vi "Read Measurement (Third Order Intercept).vi"(0 "VISA resource name":refnum<visa-resource-name>, 5 "TOI Output Format (1)":i32=1 min=0 max=2 step=1, 11 "error in (no error)":errorcluster) -> (4 "VISA resource name out":refnum<visa-resource-name>, 6 "TOI Output Format1":dbl[](array[numeric]), 8 "TOI Output Format2":T2 {"Upper_TOI" format="%.2f"; "Lower_TOI" format="%.2f"; "Worst_TOI" format="%.2f"}, 10 "TOI Output Format3":T1 {"worst_TOI" format="%.2f"; "worst_Rel" format="%.3f"; "worst_Amp" format="%.2f"; "Upper_TOI" format="%.2f"; "Upper_3rd_Rel" format="%.3f"; "Upper_3rd_Amp" format="%.2f"; "Lower_TOI" format="%.2f"; "Lower_3rd_Rel" format="%.3f"; "Upper_Tone_Amp" format="%.2f"; "Lower_Tone_Amp" format="%.2f"; "Lower_3rd_Amp" format="%.2f"}, 15 "error out":errorcluster)   [LabVIEW 2020, in "Anritsu Signal Analyzer Series.lvlib"]
doc: "Reads the measurement result of the TOI measurement."
uses:
  Anritsu Signal Analyzer Series.lvlib
panel:
  # "Frequency(Hz)"
  # "Amp(dBm)"
  # "Relative(dBc)"
  # "TOI(dBm)"
  # "Lower 3rd"
  # "Lower Tone"
  # "Upper Tone"
  # "Upper 3rd"
  # "TOI Worst"
  # "TOI(dBm)"
  # "Frequency(Hz)"
  # "Worst"
  # "Lower"
  # "Upper"
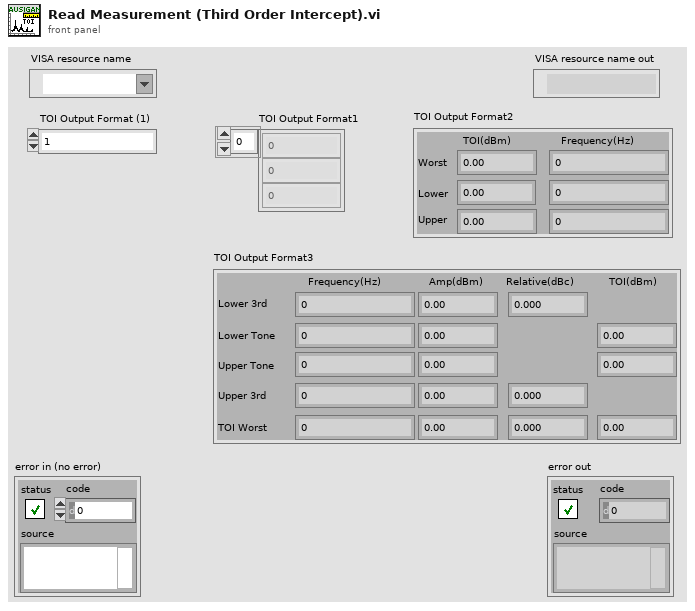
[diagram p1: front panel]
types:
  T1 = cluster{"Lower_3rd_Freq":dbl, "Lower_3rd_Amp":dbl, "Lower_3rd_Rel":dbl, "Lower_Tone_Freq":dbl, "Lower_Tone_Amp":dbl, "Lower_TOI":dbl, "Upper_Tone_Freq":dbl, "Upper_Tone_Amp":dbl, "Upper_TOI":dbl, "Upper_3rd_Freq":dbl, "Upper_3rd_Amp":dbl, "Upper_3rd_Rel":dbl, "worst_TOI_Freq":dbl, "worst_Amp":dbl, "worst_Rel":dbl, "worst_TOI":dbl}
  T2 = cluster{"Worst_TOI":dbl, "Worst_TOI_Freq":dbl, "Lower_TOI":dbl, "Lower_3rd_Freq":dbl, "Upper_TOI":dbl, "Upper_3rd_Freq":dbl}
  T3 = cluster{"Lower_3rd_Freq":dbl, "Lower_3rd_Amp":dbl, "Lower_3rd_Rel":dbl, "Lower_3rd_TOI":dbl, "Lower_Tone_Freq":dbl, "Lower_Tone_Amp":dbl, "Upper_Tone_Freq":dbl, "Upper_Tone_Amp":dbl, "Upper_3rd_Freq":dbl, "Upper_3rd_Amp":dbl, "Upper_3rd_Rel":dbl, "Upper_3rd_TOI":dbl, "worst_TOI_Freq":dbl, "worst_Amp":dbl, "worst_Rel":dbl, "worst_TOI":dbl}
  T4 = cluster{"_Default":dbl, dbl, "_Default":dbl, dbl, "_Default":dbl, dbl}
  T5 = cluster{"_Default":dbl, "_Default":dbl, "_Default":dbl, "_Default":dbl, "_Default":dbl, "_Default":dbl}
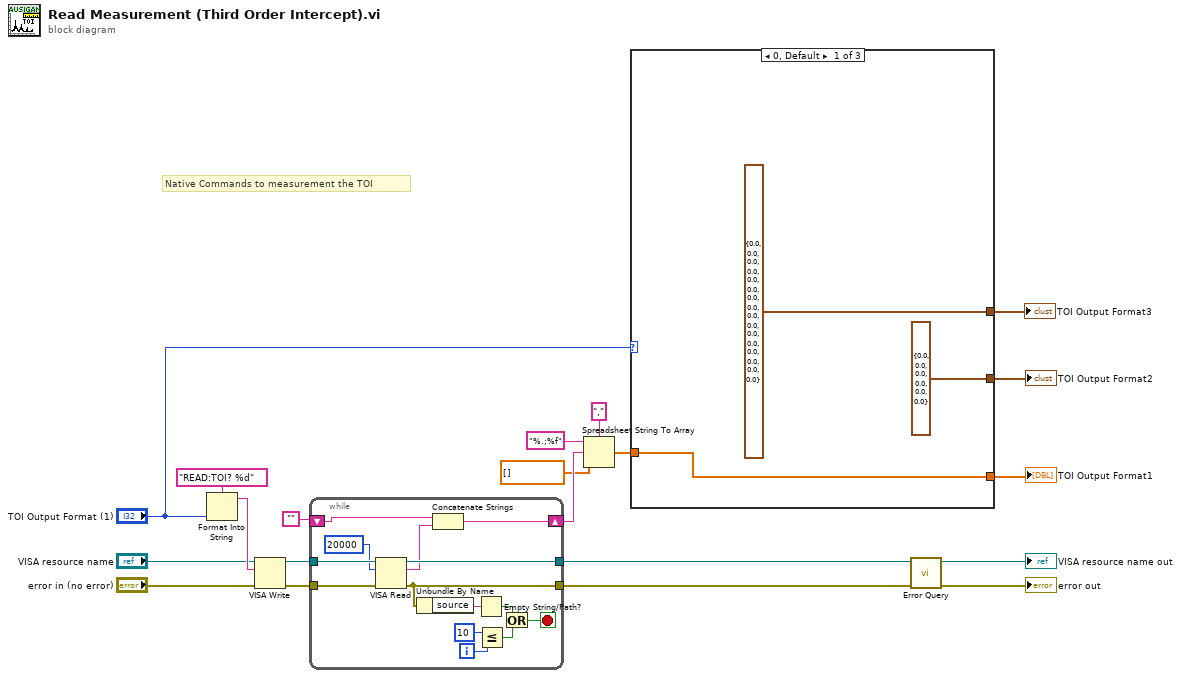
[diagram p0: block diagram]
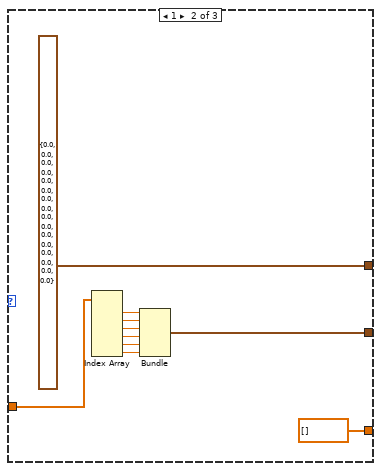
[diagram p2: hidden frame]
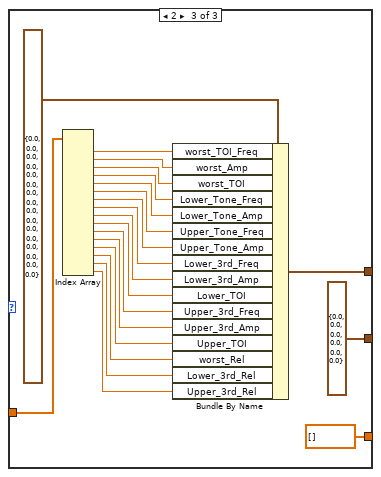
[diagram p3: hidden frame]
diagram:
  # "Native Commands to measurement the TOI"
  n1 = Format Into String(format string="READ:TOI? %d" ("_Command"), "TOI Output Format (1)") -> (resulting string=w3:string)  [unwired: 2 in, 1 out]
  n2 = VISA Write(VISA resource name="VISA resource name", write buffer=w3, error in (no error)="error in (no error)") -> (VISA resource name out=w9:refnum<visa-resource-name>, error out=w10:errorcluster)  [unwired: 1 out]
  n3 = while {
    tunnel: w9 -> [w34]
    tunnel: w10 -> [w33]
    tunnel: [w31] -> w4
    tunnel: [w30] -> w5
    shift-right: [w29] -> w11
    shift-left: "" -> [w27]
    i -> [w22]
    stop <- w26 stop-if-true
    n4 = VISA Read(VISA resource name=w34, byte count=u32 20000 ("byte count (0)"), error in (no error)=w33) -> (VISA resource name out=w31:refnum<visa-resource-name>, read buffer=w28:string, error out=w30:errorcluster)  [unwired: 1 out]
    n5 = Unbundle By Name(w30) -> ("source"=w25:string)
    n6 = Concatenate Strings(w27, w28) -> (w29:string)
    n7 = Empty String/Path?(string/path=w25) -> (empty?=w21:bool)
    n8 = Less Or Equal?(x=10, y=w22) -> (x <= y?=w24:bool)
    n9 = Or(x=w21, y=w24) -> (x .or. y?=w26:bool)
  }
  n10 = Spreadsheet String To Array(delimiter (Tab)=",", format string="%.;%f" ("Format String"), spreadsheet string=w11, array type (2D Dbl)=dbl[] []) -> (array=w14:dbl[])
  n11 = case shown="0, Default" "TOI Output Format (1)" {
    tunnel: w14 -> [w37 w46 w56]
    tunnel: [w37 dbl[] [] dbl[] []] -> w17
    tunnel: [T4 {"_Default"=0.0, 0.0, "_Default"=0.0, 0.0, "_Default"=0.0, 0.0} w42 T4 {"_Default"=0.0, 0.0, "_Default"=0.0, 0.0, "_Default"=0.0, 0.0}] -> w16
    tunnel: [T3 {"Lower_3rd_Freq"=0.0, "Lower_3rd_Amp"=0.0, "Lower_3rd_Rel"=0.0, "Lower_3rd_TOI"=0.0, "Lower_Tone_Freq"=0.0, "Lower_Tone_Amp"=0.0, "Upper_Tone_Freq"=0.0, "Upper_Tone_Amp"=0.0, "Upper_3rd_Freq"=0.0, "Upper_3rd_Amp"=0.0, "Upper_3rd_Rel"=0.0, "Upper_3rd_TOI"=0.0, "worst_TOI_Freq"=0.0, "worst_Amp"=0.0, "worst_Rel"=0.0, "worst_TOI"=0.0} ("TOI(2)") T1 {"Lower_3rd_Freq"=0.0, "Lower_3rd_Amp"=0.0, "Lower_3rd_Rel"=0.0, "Lower_Tone_Freq"=0.0, "Lower_Tone_Amp"=0.0, "Lower_TOI"=0.0, "Upper_Tone_Freq"=0.0, "Upper_Tone_Amp"=0.0, "Upper_TOI"=0.0, "Upper_3rd_Freq"=0.0, "Upper_3rd_Amp"=0.0, "Upper_3rd_Rel"=0.0, "worst_TOI_Freq"=0.0, "worst_Amp"=0.0, "worst_Rel"=0.0, "worst_TOI"=0.0} ("TOI Output Format3") w57] -> w15
    frame 0, Default {
    }
    frame 1 {
      n12 = Index Array(array=w46) -> (element #1=w45:dbl, element #2=w41:dbl, element #3=w44:dbl, element #4=w40:dbl, element #5=w43:dbl, element #6=w39:dbl)  [unwired: 6 in]
      n13 = Bundle("_Default"=w45, "_Default"=w41, "_Default"=w44, "_Default"=w40, "_Default"=w43, "_Default"=w39) -> (w42:T5)  [unwired: 1 in]
    }
    frame 2 {
      n14 = Index Array(array=w56) -> (element #1=w49:dbl, element #2=w58:dbl, element #3=w59:dbl, element #4=w50:dbl, element #5=w60:dbl, element #6=w51:dbl, element #7=w61:dbl, element #8=w52:dbl, element #9=w62:dbl, element #10=w63:dbl, element #11=w53:dbl, element #12=w64:dbl, element #13=w65:dbl, element #14=w66:dbl, element #15=w67:dbl, element #16=w68:dbl)  [unwired: 16 in]
      n15 = Bundle By Name(cluster=T1 {"Lower_3rd_Freq"=0.0, "Lower_3rd_Amp"=0.0, "Lower_3rd_Rel"=0.0, "Lower_Tone_Freq"=0.0, "Lower_Tone_Amp"=0.0, "Lower_TOI"=0.0, "Upper_Tone_Freq"=0.0, "Upper_Tone_Amp"=0.0, "Upper_TOI"=0.0, "Upper_3rd_Freq"=0.0, "Upper_3rd_Amp"=0.0, "Upper_3rd_Rel"=0.0, "worst_TOI_Freq"=0.0, "worst_Amp"=0.0, "worst_Rel"=0.0, "worst_TOI"=0.0} ("TOI Output Format3"), "worst_TOI_Freq"=w49, "worst_Amp"=w58, "worst_TOI"=w59, "Lower_Tone_Freq"=w50, "Lower_Tone_Amp"=w60, "Upper_Tone_Freq"=w51, "Upper_Tone_Amp"=w61, "Lower_3rd_Freq"=w52, "Lower_3rd_Amp"=w62, "Lower_TOI"=w63, "Upper_3rd_Freq"=w53, "Upper_3rd_Amp"=w64, "Upper_TOI"=w65, "worst_Rel"=w66, "Lower_3rd_Rel"=w67, "Upper_3rd_Rel"=w68) -> (w57:T1)
    }
  }
  "TOI Output Format1" <- w17
  "TOI Output Format2" <- w16
  "TOI Output Format3" <- w15
  n16 = call "Error Query.vi"("error in (no error)"=w5, "VISA resource name"=w4) -> ("error out"=→"error out":errorcluster, "VISA resource name out"=→"VISA resource name out":refnum<visa-resource-name>)  [unwired: 6 in, 2 out]
